vi "Color Change.vi"(10 "Alpha":dbl=1.0, 11 "Color":u32(colorbox)) -> (3 "RGBA":cluster{"R":sgl, "G":sgl, "B":sgl, "A":sgl})   [LabVIEW 2020, in "NI_3D Picture Control.lvlib"]
doc: "Converts an RGB color and an alpha into an RGBA cluster that you can apply to a 3D object."
uses:
  NI_3D Picture Control.lvlib
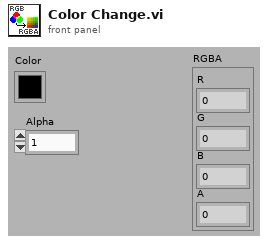
[diagram p1: front panel]
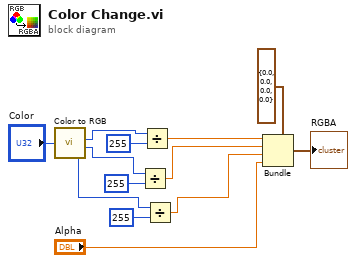
[diagram p0: block diagram]
diagram:
  n1 = call "Color to RGB.vi"("Color"="Color") -> ("R"=w8:u8, "G"=w7:u8, "B"=w6:u8)  [unwired: 1 out]
  n2 = Divide(x=w7, y=u32 255) -> (x/y=w3:dbl)
  n3 = Divide(x=w8, y=u32 255) -> (x/y=w4:dbl)
  n4 = Divide(x=w6, y=u32 255) -> (x/y=w2:dbl)
  n5 = Bundle(cluster=cluster{"R":sgl, "G":sgl, "B":sgl, "B":sgl} {"R"=0.0, "G"=0.0, "B"=0.0, "B"=0.0}, "R"=w4, "G"=w3, "B"=w2, "B"="Alpha") -> (→"RGBA":cluster{"R":sgl, "G":sgl, "B":sgl, "B":sgl})
